vi "Host.vi"   [LabVIEW 2025]
uses:
  <vilib>/Handler Framework/Handler Framework.lvlib
  <vilib>/Handler Framework/CmdQueue/Enqueue Single.vi
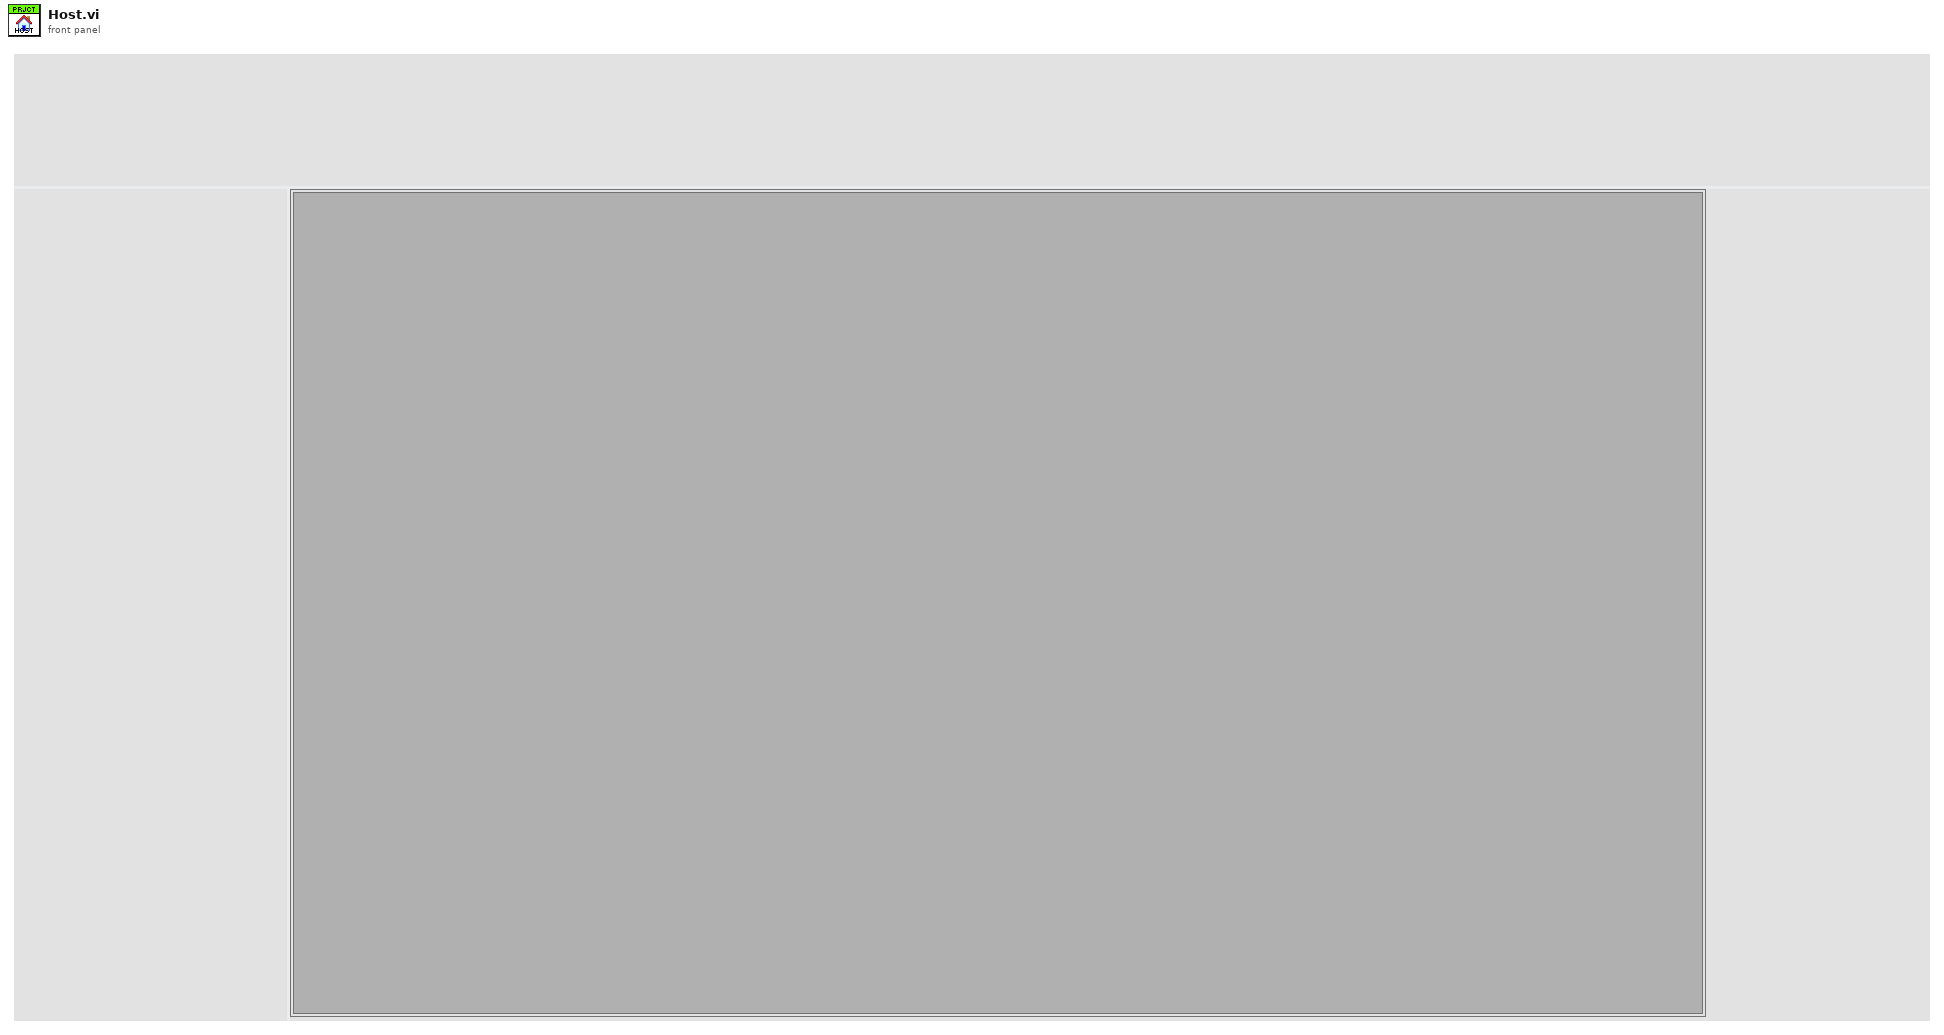
[diagram p1: front panel]
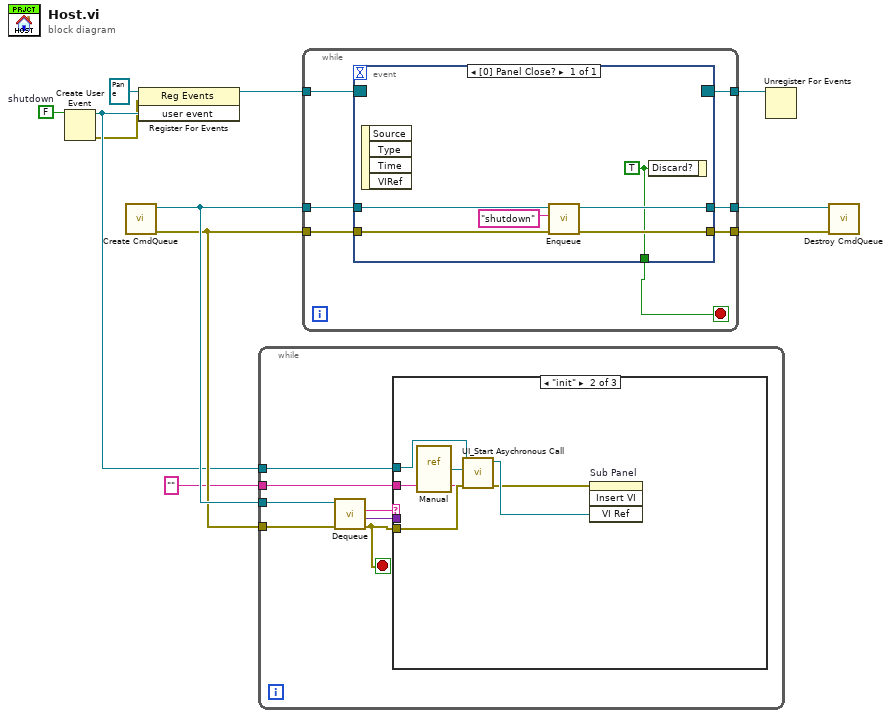
[diagram p0: block diagram]
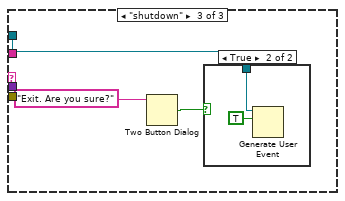
[diagram p3: hidden frame]
diagram:
  w7 = FALSE  # shutdown
  n1 = Create User Event(user event datatype=w7) -> (user event=w4:refnum<user-event>, error out=w1:errorcluster)  [unwired: 1 in]
  n2 = call <vilib>:"Create CmdQueue.vi"() -> ("error out"=w8:errorcluster, "CmdQueue out"=w9:refnum<queue>)  [unwired: 10 in]
  n3 = register-events(reference=refnum<event-registration> refnum ("event registration refnum"), error in=w1, w4) -> (reference out=w6:refnum<event-registration>)  [unwired: 1 out]
  n4 = while {
    tunnel: w9 -> [w18]
    tunnel: w8 -> [w15]
    tunnel: w4 -> [w14]
    tunnel: "" ("String") -> [w12]
    stop <- w13 stop-if-true
    n5 = call <vilib>:"Dequeue.vi"("error in (no error)"=w15, "CmdQueue in"=w18) -> ("error out"=w13:errorcluster, "value"=w16:variant, "cmd"=w17:string)  [unwired: 5 in, 2 out]
    n6 = case shown="\"init\"" w17 {
      tunnel: w16 -> [_ _ _]
      tunnel: w14 -> [_ w20 w25]
      tunnel: w13 -> [_ w21 _]
      tunnel: w12 -> [_ w19 _]
      frame "False", Default {
      }
      frame "init" {
        n7 = vi-ref "Manual.vi"() -> (w24:refnum<vi>)
        n8 = call "UI_Start Asychronous Call.vi"("error in (no error)"=w21, "String"=w19, "VI Refnum"=w24, "User Event in"=w20) -> ("error out"=w22:errorcluster, "VI out"=w23:refnum<vi>)  [unwired: 6 in]
        n9 = invoke on="Sub Panel" class="SubPnl" method="Insert VI"(error in=w22, "VI Ref"=w23) -> ()  [unwired: 2 in, 4 out]
      }
      frame "shutdown" {
        n10 = Two Button Dialog(message="Exit. Are you sure?") -> (T button?=w26:bool)  [unwired: 2 in]
        n11 = case shown="True" w26 {
          tunnel: w25 -> [_ w29]
          frame False {
          }
          frame True {
            n12 = Generate User Event(user event=w29, event data cluster=TRUE ("event data")) -> ()  [unwired: 2 in, 2 out]
          }
        }
      }
    }
  }
  n13 = while {
    tunnel: w9 -> [w34]
    tunnel: [w32] -> w11
    tunnel: w8 -> [w33]
    tunnel: [w31] -> w10
    tunnel: w6 -> [w36]
    tunnel: [w35] -> w5
    stop <- w30 stop-if-true
    n14 = event shown="[0] Panel Close?" {
      selector: w36 -> [_]
      dyn-events: [_] -> w35
      timeout: _ -> [_]
      tunnel: w34 -> [w41]
      tunnel: w33 -> [w40]
      tunnel: [w39] -> w32
      tunnel: [w38] -> w31
      tunnel: [w37] -> w30
      event Panel Close? {
        w37 = TRUE ("Discard?")
        n15 = event-data() -> ()  [unwired: 1 in, 4 out]
        n16 = call-poly <vilib>:"Enqueue.vi"("error in (no error)"=w40, "Command"="shutdown", "CmdQueue in"=w41) -> ("error out"=w38:errorcluster, "CmdQueue out"=w39:refnum<queue>)  [unwired: 7 in]
        n17 = event-data("Discard?"=w37) -> ()  [unwired: 1 in, 1 out]
      }
    }
  }
  n18 = Unregister For Events(event registration refnum=w5) -> ()  [unwired: 1 in, 1 out]
  n19 = call <vilib>:"Destroy CmdQueue.vi"("error in (no error)"=w10, "CmdQueue in"=w11) -> ()  [unwired: 9 in, 1 out]
